vi "Read File Path Control.vi"(8 "error in (no error)":errorcluster, 11 "Load Functions Message in":refnum<class "Find Functions On Disk Message.lvclass">) -> (0 "error out":errorcluster, 2 "Array of Function Paths":path[](array[path]), 3 "Load Functions Message out":refnum<class "Find Functions On Disk Message.lvclass">)   [LabVIEW 2016, in "Controller Actor.lvlib" / "Find Functions On Disk Message.lvclass"]
uses:
  <userlib>/Common Components/Controller/Messages/Load Functions/Find Functions On Disk Message.lvclass
  <userlib>/Common Components/Controller/Messages/Load Functions/Find Functions On Disk Message.lvclass/Find Functions On Disk Message.ctl
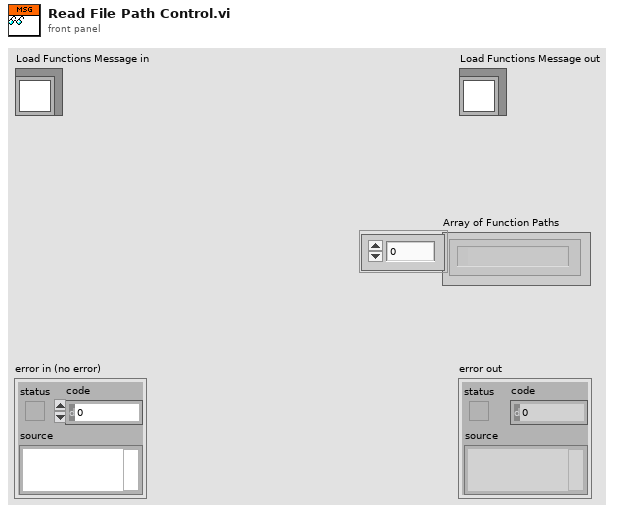
[diagram p1: front panel]
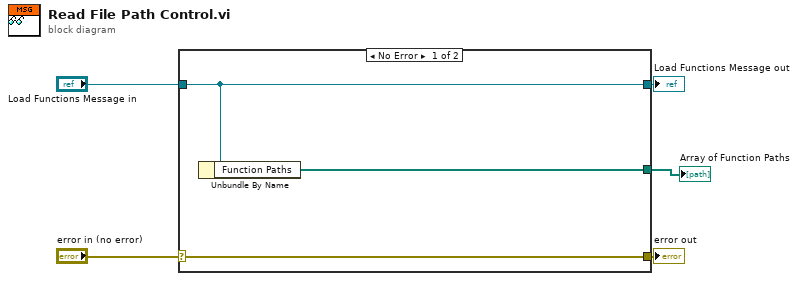
[diagram p0: block diagram]
diagram:
  n1 = case shown="No Error" "error in (no error)" {
    selector: "error in (no error)" -> [w8 w9]
    tunnel: [w8 w9] -> w4
    tunnel: [w7 w10] -> w2
    tunnel: "Load Functions Message in" -> [w7 w10]
    tunnel: [w6 _] -> w1
    frame No Error {
      n2 = Unbundle By Name(w7) -> ("Function Paths"=w6:path[])
    }
    frame Error {
    }
  }
  "error out" <- w4
  "Load Functions Message out" <- w2
  "Array of Function Paths" <- w1
